vi "Apply Configuration.vi"(8 "Error In":errorcluster, 11 "reference in":refnum<class "Instrument.lvclass">) -> (0 "Error Out":errorcluster, 3 "reference out":refnum<class "Instrument.lvclass">)   [LabVIEW 2023, in "HAL GOOP4.lvlib" / "Instrument.lvclass"]
uses:
  Instrument.lvclass
  Instrument.lvclass/Instrument.ctl
  Interfaces/IConfigure/IConfigure.lvclass
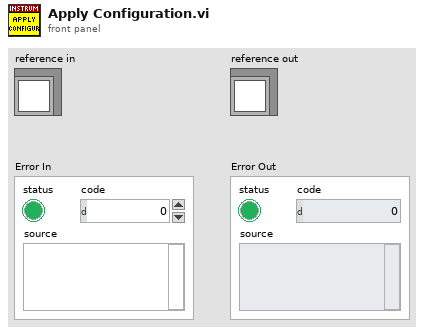
[diagram p1: front panel]
types:
  T1 = typedef "HAL GOOP4.lvlib/Instrument.lvclass/ObjectAttributes.ctl" = cluster{"IConfigure":refnum<class "IConfigure.lvclass">, "Ref Count":u8, "Start Count":u8}
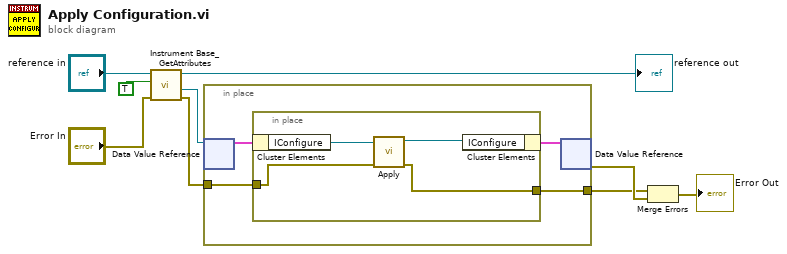
[diagram p0: block diagram]
diagram:
  n1 = call "Instrument Base_GetAttributes.vi"("Error In"="Error In", "OnlyGetDvrReference(False)"=TRUE, "reference in"="reference in") -> ("Error Out"=w3:errorcluster, "DataRef"=w4:refnum<data-value>, "reference out"=→"reference out":refnum<class "Instrument.lvclass">)  [unwired: 5 in, 1 out]
  n2 = in-place {
    in-place-border: w3 -> [w11]
    in-place-border: [w10] -> w1
    n3 = in-place-dvr #1(w4) -> (w13:T1)  [unwired: 1 out]
    n4 = in-place {
      in-place-border: w11 -> [w15]
      in-place-border: [w14] -> w10
      n5 = in-place-cluster #2(w13) -> ("IConfigure"=w17:refnum<class "IConfigure.lvclass">)
      n6 = call-dynamic "Apply.vi"("error in (no error)"=w15, "IConfigure in"=w17) -> ("error out"=w14:errorcluster, "IConfigure out"=w16:refnum<class "IConfigure.lvclass">)  [unwired: 8 in]
      n7 = in-place-cluster #2("IConfigure"=w16) -> (w12:T1)
    }
    n8 = in-place-dvr #1(w12) -> (w2:errorcluster)  [unwired: 1 out]
  }
  n9 = Merge Errors(w1, w2) -> (→"Error Out":errorcluster)
